vi "抓圓.vi"(0 "Image In":T2, 1 "Process":T7(ring), 2 "Optimized Mode":bool, 3 "Direction":enum16{"Inner to Outer", "Outer to Inner"}(ring), 5 "ROI":T1, 9 "Gap":i32=10 min=1 max=300, 11 "error In":errorcluster, 12 "Edge Options":T5={"Edge Polarity"=0, "Kernel Size"=3, "Width"=3, "Minimum Edge Strength"=10.0, "Interpolation Type"=enum."Bilinear Fixed", "Data Processing Method"=enum."Average"} {"Edge Polarity" items=["All Edges", "Rising Edges", "Falling Edges"]; "Minimum Edge Strength" format="%.2f"; "Width" step=2; "Kernel Size" step=2}, 13 "Point Diameter (5)":u32=5 min=3 max=1000) -> (4 "Imag e Out":T2, 6 "Line Profile":T3(graph), 10 "Gradient Information":dbl[][](graph), 14 "Ellipse":T4 {"Minor Axis"."Point 2"."Y" format="%.2f"; "Minor Axis"."Point 2"."X" format="%.2f"; "Minor Axis"."Point 1"."Y" format="%.2f"; "Minor Axis"."Point 1"."X" format="%.2f"; "Major Axis"."Point 2"."Y" format="%.2f"; "Major Axis"."Point 2"."X" format="%.2f"; "Major Axis"."Point 1"."Y" format="%.2f"; "Major Axis"."Point 1"."X" format="%.2f"; "Center"."Y" format="%.2f"; "Center"."X" format="%.2f"}, 15 "error out":errorcluster)   [LabVIEW 2015]
uses:
  <vilib>/vision/Measure.llb/Edge Options.ctl
  <vilib>/vision/Measure.llb/Edge Polarity.ctl
  <vilib>/vision/Image Controls.llb/IMAQ Image.ctl
  <vilib>/Analysis/coordinate.llb/2D Cartesian Coordinate Rotation (Scalar).vi
  <vilib>/vision/NI_Vision_Development_Module.lvlib
  <vilib>/Analysis/NI_AALPro.lvlib
panel:
  out "error out 2":errorcluster
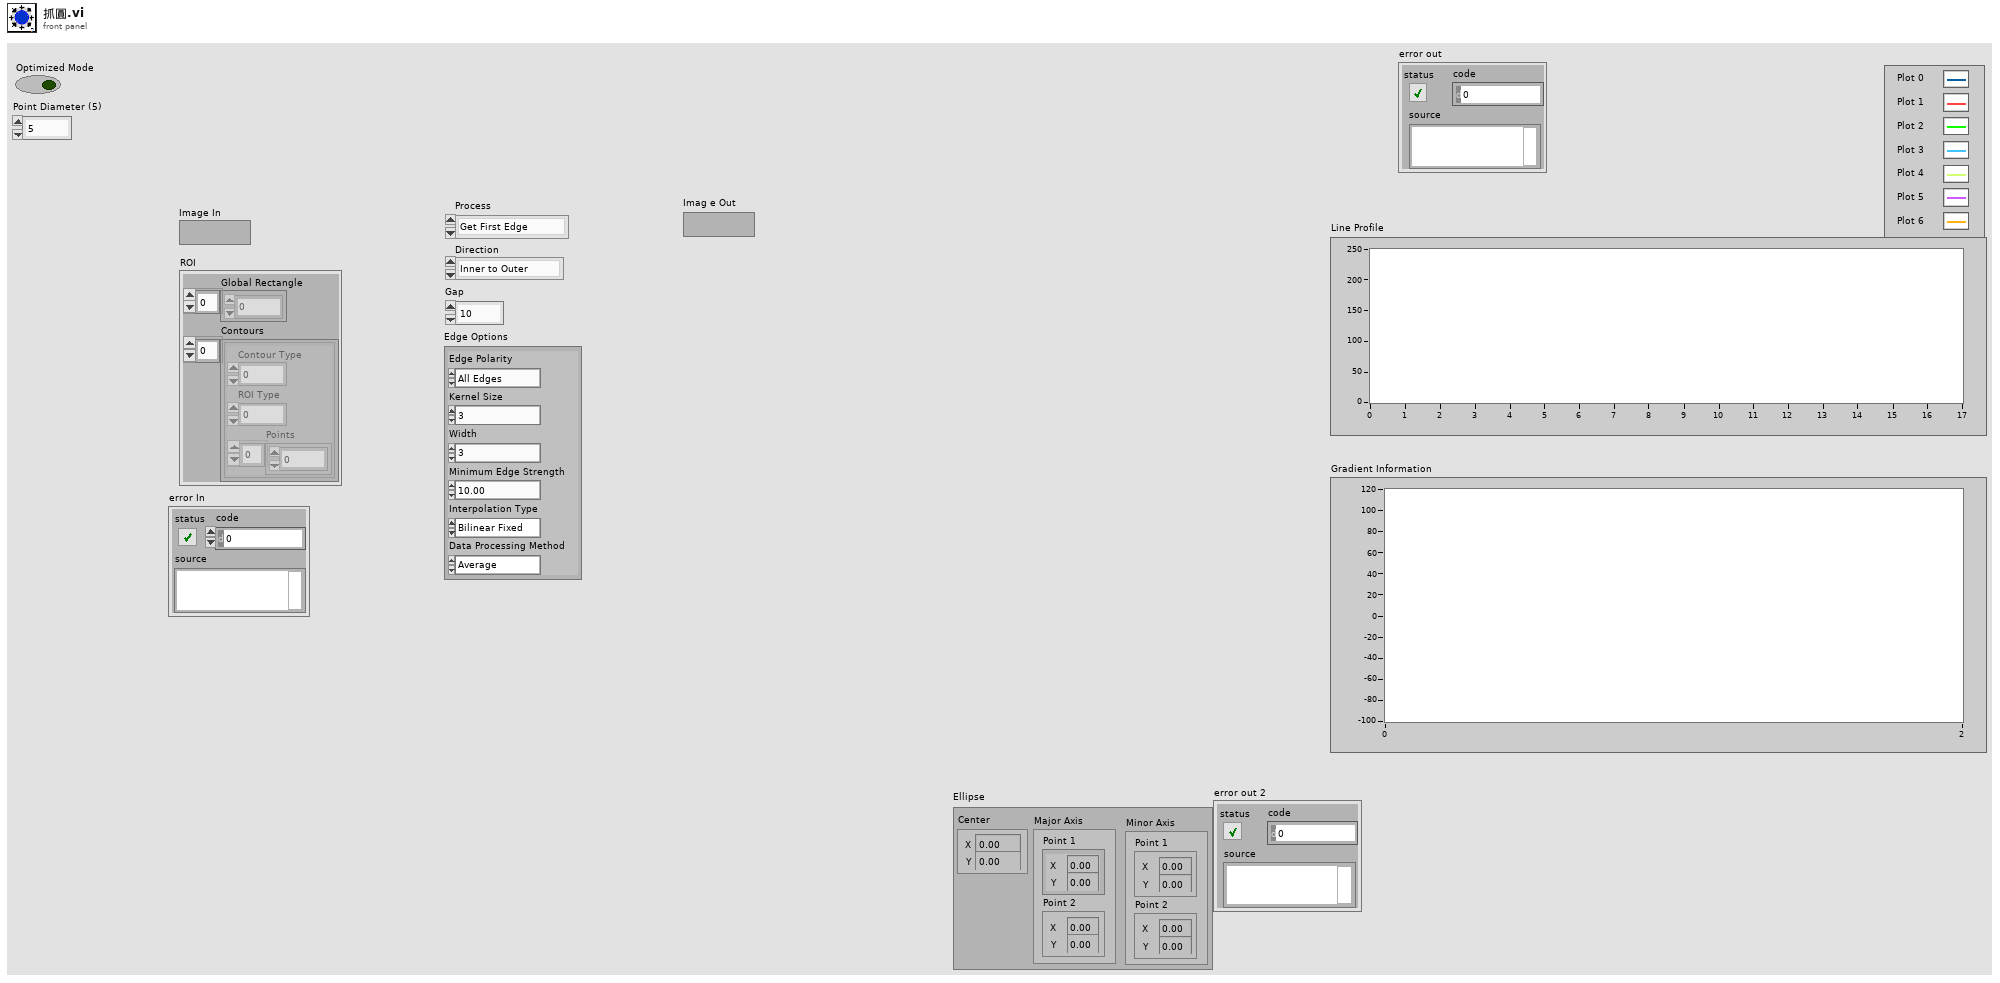
[diagram p1: front panel]
types:
  T1 = cluster{"Global Rectangle":i32[], "Contours":cluster{"Contour Type":u32, "ROI Type":u32, "Points":i32[]}[]}
  T2 = typedef "IMAQ Image.ctl" = refnum<image>
  T3 = cluster{"x0":sgl, "dx":sgl, "Pixels Line":sgl[]}[]
  T4 = cluster{"Center":cluster{"X":sgl, "Y":sgl}, "Major Axis":cluster{"Point 1":cluster{"X":sgl, "Y":sgl}, "Point 2":cluster{"X":sgl, "Y":sgl}}, "Minor Axis":cluster{"Point 1":cluster{"X":sgl, "Y":sgl}, "Point 2":cluster{"X":sgl, "Y":sgl}}}
  T5 = typedef "Edge Options.ctl" = cluster{"Edge Polarity":T6, "Kernel Size":u32, "Width":u32, "Minimum Edge Strength":sgl, "Interpolation Type":enum32{"Zero Order", "Bilinear", "Quadratic", "Cubic", "Bilinear Fixed"}, "Data Processing Method":enum32{"Average", "Median"}}
  T6 = typedef "Edge Polarity.ctl" = u32
  T7 = enum16{"Get First Edge", "Get First + Last Edge", "Get All Edges", "Get Best Edge"}
  T8 = typedef "IMAQ Point" = cluster{"X":sgl, "Y":sgl}
  T9 = typedef "IMAQ Circle" = cluster{"Center X":i32, "Center Y":i32, "Inner Radius":i32, "Outer Radius":i32, "Start Angle":dbl, "End Angle":dbl}
  T10 = cluster{"Point 1":cluster{"x":dbl, "y":dbl}, "Point 2":cluster{"x":dbl, "y":dbl}}
  T11 = typedef "IMAQ Line" = cluster{"Start X":i32, "Start Y":i32, "End X":i32, "End Y":i32}
  T12 = typedef "ROI Descriptor" = cluster{"Global Rectangle":i32[], "Contours":cluster{"ID":enum32{"External", "Internal"}, "Type":u32, "Coordinates":i32[]}[]}
  T13 = typedef "Edge New.ctl" = cluster{"Location (Pixel)":cluster{"X":sgl, "Y":sgl}, "Location (Real-World)":cluster{"X":sgl, "Y":sgl}, "Distance (Pixel)":dbl, "Distance (Real-World)":dbl, "Strength":dbl, "Noise":dbl, "Rising?":bool}
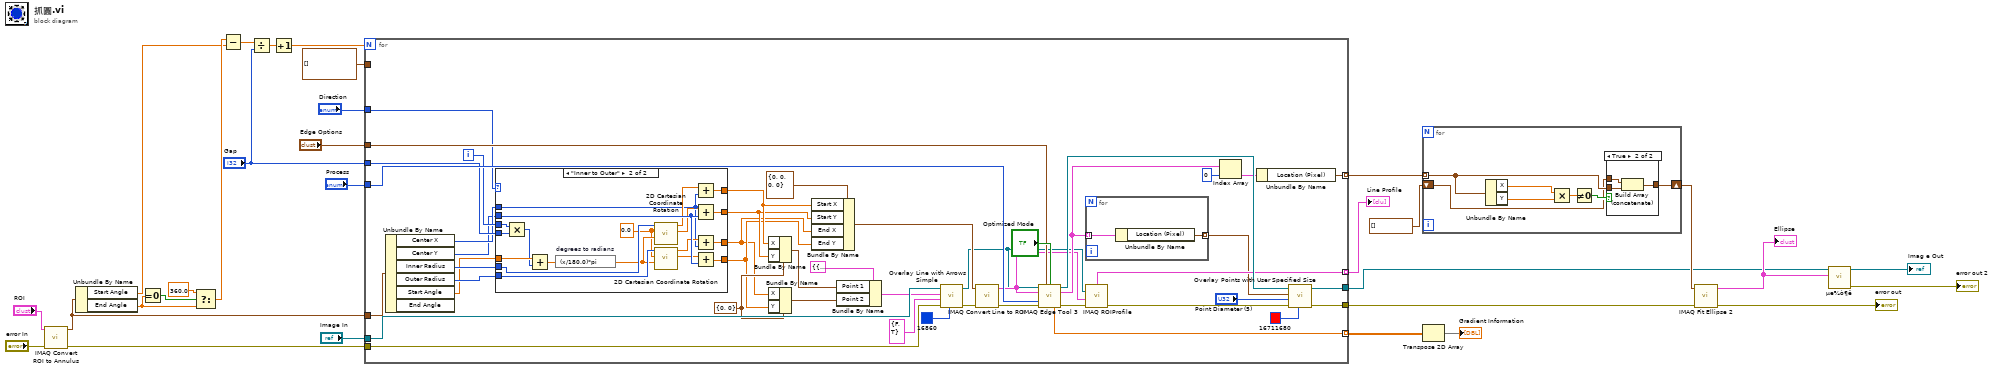
[diagram p0: block diagram]
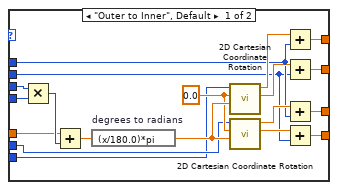
[diagram p3: hidden frame]
diagram:
  n1 = call "IMAQ Convert ROI to Annulus"("error in (no error)"="error In", "ROI Descriptor"="ROI") -> ("error out"=w23:errorcluster, "Annulus"=w18:T9)  [unwired: 7 in]
  n2 = Unbundle By Name(w18) -> ("Start Angle"=w8:dbl, "End Angle"=w9:dbl)
  n3 = Equal To 0?(x=w9) -> (x = 0?=w14:bool)
  n4 = Select(t=360.0, s=w14, f=w9) -> (s? t:f=w12:dbl)
  n5 = Subtract(x=w12, y=w8) -> (x-y=w11:dbl)
  n6 = Divide(x=w11, y="Gap") -> (x/y=w10:dbl)
  n7 = Increment(x=w10) -> (x+1=w24:dbl)
  n8 = for {
    N: w24 -> [_]
    tunnel: "Direction" -> [w60]
    tunnel: [w70] -> w3
    tunnel: "Image In" -> [w61]
    tunnel: w23 -> [w58]
    tunnel: [w69] -> w19
    tunnel: "Process" -> [w71]
    tunnel: "Edge Options" -> [w68]
    tunnel: [w67] -> w22 mode=indexing
    tunnel: [w66] -> w25 mode=indexing
    tunnel: [w65] -> w21 mode=indexing
    tunnel: "Gap" -> [w57]
    tunnel: w18 -> [w55]
    tunnel: T8[] [] ("Rectangle Points") -> [_]
    i -> [w56]
    w52 = cluster{"X":i32, "Y":i32} {"X"=0, "Y"=0} ("Start Point")
    n9 = Unbundle By Name(w55) -> ("Center X"=w36:i32, "Center Y"=w35:i32, "Inner Radius"=w34:i32, "Outer Radius"=w33:i32, "Start Angle"=w32:dbl)  [unwired: 1 out]
    n10 = case shown="\"Inner to Outer\"" w60 {
      tunnel: w35 -> [w78 w113]
      tunnel: w34 -> [w77 w112]
      tunnel: w33 -> [w76 w111]
      tunnel: w32 -> [w81 w110]
      tunnel: w57 -> [w79 w109]
      tunnel: w56 -> [w80 w100]
      tunnel: [w86 w95] -> w44
      tunnel: [w84 w99] -> w42
      tunnel: w36 -> [w82 w98]
      tunnel: [w83 w97] -> w41
      tunnel: [w85 w96] -> w43
      frame "Outer to Inner", Default {
        w89 = 0.0 ("y")
        n11 = Multiply(x=w80, y=w79) -> (x*y=w88:i32)
        n12 = Add(x=w81, y=w88) -> (x+y=w87:dbl)
        n13 = expression code="(x/180.0)*pi" "degrees to radians"(w87) -> (w90:dbl)
        n14 = call-poly <vilib>:"2D Cartesian Coordinate Rotation.vi"("theta"=w90, "y"=w89, "x"=w76) -> ("y out"=w93:dbl, "x out"=w94:dbl)  [unwired: 6 in, 1 out]
        n15 = call-poly <vilib>:"2D Cartesian Coordinate Rotation.vi"("theta"=w90, "y"=w89, "x"=w77) -> ("y out"=w92:dbl, "x out"=w91:dbl)  [unwired: 6 in, 1 out]
        n16 = Add(x=w94, y=w82) -> (x+y=w86:dbl)
        n17 = Add(x=w93, y=w78) -> (x+y=w85:dbl)
        n18 = Add(x=w91, y=w82) -> (x+y=w83:dbl)
        n19 = Add(x=w92, y=w78) -> (x+y=w84:dbl)
      }
      frame "Inner to Outer" {
        w103 = 0.0 ("y")
        n20 = Multiply(x=w100, y=w109) -> (x*y=w102:i32)
        n21 = Add(x=w110, y=w102) -> (x+y=w101:dbl)
        n22 = expression code="(x/180.0)*pi" "degrees to radians"(w101) -> (w104:dbl)
        n23 = call-poly <vilib>:"2D Cartesian Coordinate Rotation.vi"("theta"=w104, "y"=w103, "x"=w112) -> ("y out"=w107:dbl, "x out"=w108:dbl)  [unwired: 6 in, 1 out]
        n24 = call-poly <vilib>:"2D Cartesian Coordinate Rotation.vi"("theta"=w104, "y"=w103, "x"=w111) -> ("y out"=w106:dbl, "x out"=w105:dbl)  [unwired: 6 in, 1 out]
        n25 = Add(x=w108, y=w98) -> (x+y=w95:dbl)
        n26 = Add(x=w107, y=w113) -> (x+y=w96:dbl)
        n27 = Add(x=w105, y=w98) -> (x+y=w97:dbl)
        n28 = Add(x=w106, y=w113) -> (x+y=w99:dbl)
      }
    }
    n29 = Bundle By Name(cluster=w52, "X"=w44, "Y"=w43) -> (w50:cluster{"X":i32, "Y":i32})
    n30 = Bundle By Name(cluster=w52, "X"=w41, "Y"=w42) -> (w51:cluster{"X":i32, "Y":i32})
    n31 = Bundle By Name(cluster=T11 {"Start X"=0, "Start Y"=0, "End X"=0, "End Y"=0} ("Line"), "Start X"=w44, "Start Y"=w43, "End X"=w41, "End Y"=w42) -> (w53:T11)
    n32 = Bundle By Name(cluster=T10 {"Point 1"={"x"=50.0, "y"=50.0}, "Point 2"={"x"=70.0, "y"=70.0}} ("Line Coordinates"), "Point 1"=w50, "Point 2"=w51) -> (w47:T10)
    n33 = call "Overlay Line with Arrows Simple.vi"("Color"=u32 16860, "error in"=w58, "Arrows"=cluster{"Start point":bool, "End point":bool} {"Start point"=FALSE, "End point"=TRUE}, "Line Coordinates"=w47, "Image In"=w61) -> ("error out"=w45:errorcluster, "Image Out"=w46:T2)  [unwired: 5 in]
    n34 = call "IMAQ Convert Line to ROI"("error in (no error)"=w45, "Line"=w53) -> ("error out"=w63:errorcluster, "ROI Descriptor"=w62:T12)  [unwired: 7 in]
    n35 = call "IMAQ Edge Tool 3"("Image"=w46, "Edge Options"=w68, "Optimized Mode"="Optimized Mode", "ROI Descriptor"=w62, "Process"=w71, "error in (no error)"=w63) -> ("Image (duplicate)"=w72:T2, "Edge Information"=w75:T13[], "Gradient Values"=w66:dbl[], "error out"=w64:errorcluster)  [unwired: 5 in, 1 out]
    n36 = for {
      tunnel: w75 -> [w115] mode=indexing
      tunnel: [w114] -> w37 mode=indexing
      n37 = Unbundle By Name(w115) -> ("Location (Pixel)"=w114:cluster{"X":sgl, "Y":sgl})
    }
    n38 = call "IMAQ ROIProfile"("error in (no error)"=w64, "ROI Descriptor"=w62, "Image"=w46) -> ("error out"=w74:errorcluster, "ROI Graph"=w67:cluster{"x0":sgl, "dx":sgl, "Pixels Line":sgl[]})  [unwired: 1 in, 3 out]
    n39 = Index Array(array=w75, index=0) -> (element=w38:T13)
    n40 = Unbundle By Name(w38) -> ("Location (Pixel)"=w65:cluster{"X":sgl, "Y":sgl})
    n41 = call "Overlay Points with User Specified Size.vi"("Color"=u32 16711680, "error in"=w74, "Point Diameter (5)"="Point Diameter (5)", "Points"=w37, "Image In"=w72) -> ("error out"=w69:errorcluster, "Image Out"=w70:T2)  [unwired: 5 in]
  }
  "Line Profile" <- w22
  n42 = for {
    tunnel: w21 -> [w118] mode=indexing
    shift-right: [w117] -> w20
    shift-left: cluster{"X":sgl, "Y":sgl}[] [] -> [w116]
    n43 = Unbundle By Name(w118) -> ("X"=w122:sgl, "Y"=w121:sgl)
    n44 = Multiply(x=w122, y=w121) -> (x*y=w120:sgl)
    n45 = Not Equal To 0?(x=w120) -> (x != 0?=w119:bool)
    n46 = case shown="True" w119 {
      tunnel: w118 -> [_ w126]
      tunnel: [w123 w125] -> w117
      tunnel: w116 -> [w123 w124]
      frame False {
      }
      frame True {
        n47 = Build Array (concatenate)(w124, w126) -> (w125:cluster{"X":sgl, "Y":sgl}[])
      }
    }
  }
  n48 = Transpose 2D Array(2D array=w25) -> (transposed array=→"Gradient Information":dbl[][])
  n49 = call "IMAQ Fit Ellipse 2"("error in (no error)"=w19, "Radial Points"=w20) -> ("error out"=→"error out":errorcluster, "Ellipse"=w4:T4)  [unwired: 4 in, 4 out]
  "Ellipse" <- w4
  n50 = call "µe¾ò¶ê.vi"("Ellipse"=w4, "Image In"=w3) -> ("error out"=→"error out 2":errorcluster, "Image"=→"Imag e Out":T2)  [unwired: 8 in]
